vi "UartCom.vi"(1 "String":string="head b", 2 "VISA resource name":refnum<visa-resource-name>="COM4") -> (0 "read buffer":string)   [LabVIEW 2014]
uses:
  <vilib>/Instr/_visa.llb/VISA Configure Serial Port (Instr).vi
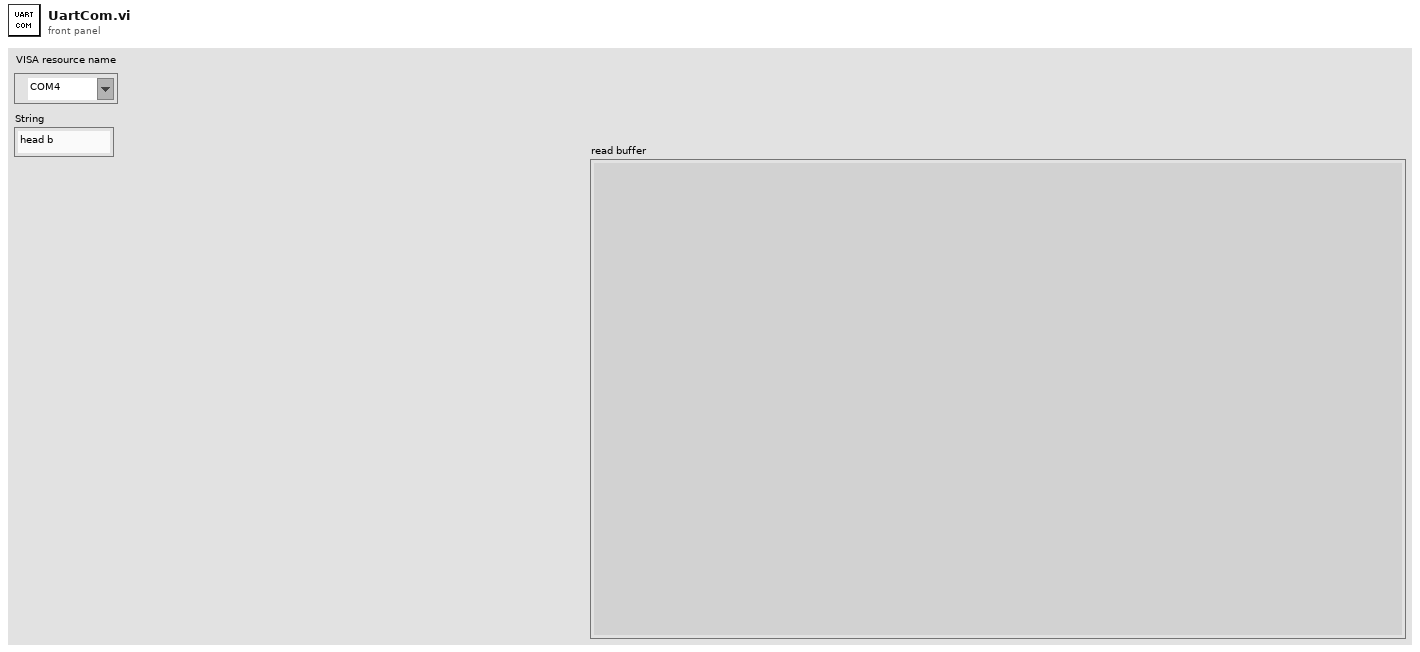
[diagram p1: front panel]
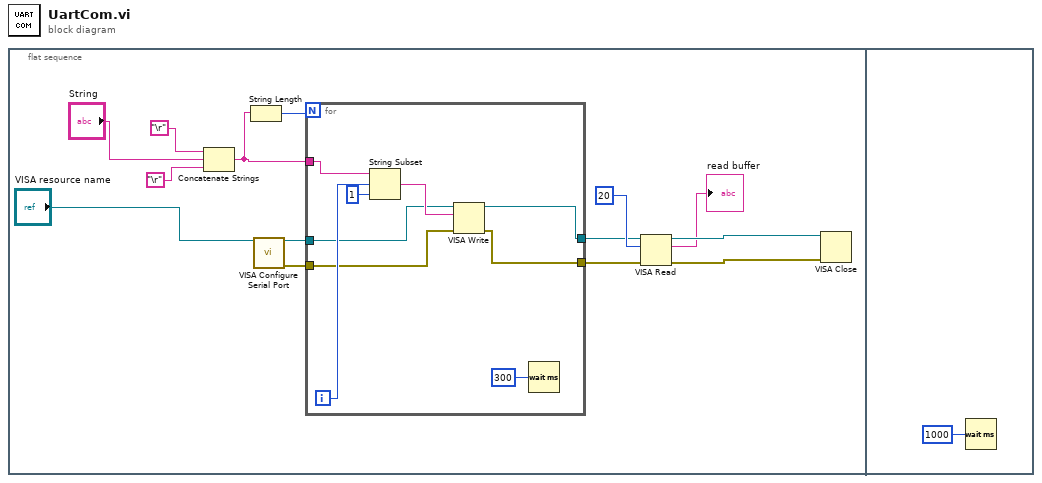
[diagram p0: block diagram]
diagram:
  n1 = flat-sequence {
    frame #0 {
      n2 = Concatenate Strings("\r", "String", "\r") -> (w5:string)
      n3 = String Length(string=w5) -> (length=w6:i32)
      n4 = call-poly "VISA Configure Serial Port"("VISA resource name"="VISA resource name") -> ("VISA resource name out"=w2:refnum<visa-resource-name>, "error out"=w1:errorcluster)  [unwired: 13 in]
      n5 = for {
        N: w6 -> [_]
        tunnel: w5 -> [w21]
        tunnel: [w19] -> w4
        tunnel: [w18] -> w3
        tunnel: w2 -> [w17]
        tunnel: w1 -> [w16]
        i -> [w23]
        n6 = String Subset(string=w21, offset (0)=w23, length (rest)=1 ("length (rest)")) -> (substring=w20:string)
        n7 = VISA Write(VISA resource name=w17, write buffer=w20, error in (no error)=w16) -> (VISA resource name out=w18:refnum<visa-resource-name>, error out=w19:errorcluster)  [unwired: 1 out]
        n8 = Wait (ms)(milliseconds to wait=u32 300) -> ()  [unwired: 1 out]
      }
      n9 = VISA Read(VISA resource name=w3, byte count=u32 20, error in (no error)=w4) -> (VISA resource name out=w13:refnum<visa-resource-name>, read buffer=→"read buffer":string, error out=w12:errorcluster)  [unwired: 1 out]
      n10 = VISA Close(VISA resource name=w13, error in (no error)=w12) -> ()  [unwired: 1 out]
    }
    frame #1 {
      n11 = Wait (ms)(milliseconds to wait=u32 1000) -> ()  [unwired: 1 out]
    }
  }
